vi "K8055.vi"() -> (0 "Numeric":dbl)   [LabVIEW 2012]
uses:
  K8055D.dll
panel:
  in  "Card":dbl
  out "Numeric 2":dbl
  in  "Knob 2":dbl(knob) min=0.0 max=255.0 step=1.0 scale=0.0..255.0
  in  "Knob":dbl(knob) max=255.0 step=1.0 scale=0.0..255.0
  out "Boolean 13":bool
  out "Boolean 12":bool
  out "Boolean 11":bool
  out "Boolean 10":bool
  out "Boolean 9":bool
  in  "Boolean 8":bool
  in  "Boolean 7":bool
  in  "Boolean 6":bool
  in  "Boolean 5":bool
  in  "Boolean 4":bool
  in  "Boolean 3":bool
  in  "Boolean 2":bool
  in  "Boolean":bool
  # "Driver for Velleman K8055 board\nproblems?  email  mike.rendall@gmail.com"
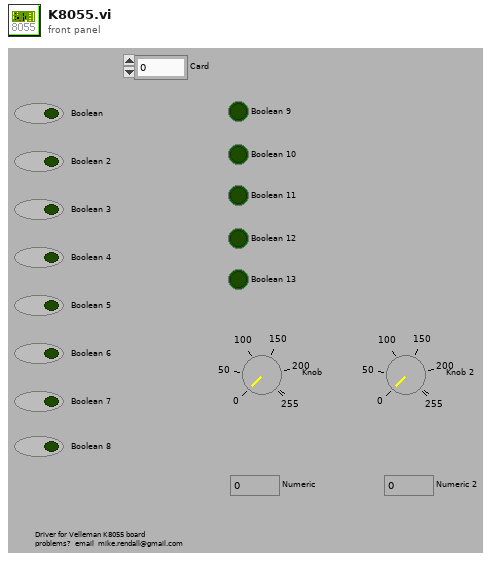
[diagram p1: front panel]
types:
  T1 = cluster{"Boolean array[0]":bool, "Boolean array[1]":bool, "Boolean array[2]":bool, "Boolean array[3]":bool, "Boolean array[4]":bool, "Boolean array[5]":bool, "Boolean array[6]":bool, "Boolean array[7]":bool, "Boolean array[8]":bool}
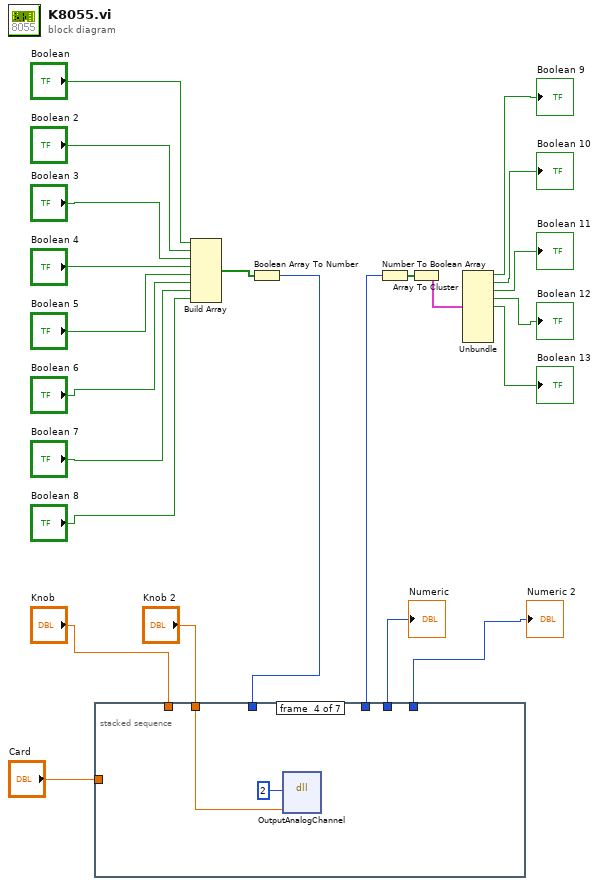
[diagram p0: block diagram]
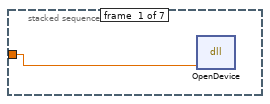
[diagram p2: hidden frame]
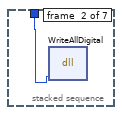
[diagram p3: hidden frame]
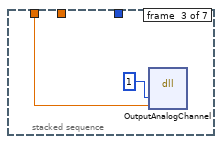
[diagram p4: hidden frame]
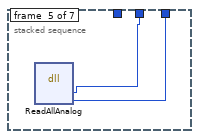
[diagram p5: hidden frame]
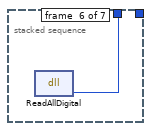
[diagram p6: hidden frame]
diagram:
  n1 = Build Array("Boolean", "Boolean 2", "Boolean 3", "Boolean 4", "Boolean 5", "Boolean 6", "Boolean 7", "Boolean 8") -> (w15:bool[])
  n2 = Boolean Array To Number(Boolean array=w15) -> (number=w13:u32)
  n3 = stacked-sequence {
    tunnel: "Card" -> [w24 _ _ _ _ _ _]
    tunnel: w13 -> [_ w25 _ _ _ _ _]
    tunnel: "Knob" -> [_ _ w27 _ _ _ _]
    tunnel: "Knob 2" -> [_ _ _ w29 _ _ _]
    tunnel: [_ _ _ _ w31 _ _] -> w10
    tunnel: [_ _ _ _ w30 _ _] -> w9
    tunnel: [_ _ _ _ _ w32 _] -> w8
    frame #0 {
      n4 = dll-call lib="C:/Users/edm/Desktop/experiment control/subvis/USB DAQ/K8055D.dll" fn="OpenDevice"(w24) -> ()  [unwired: 5 in, 2 out]
    }
    frame #1 {
      n5 = dll-call lib="C:/Users/edm/Desktop/experiment control/subvis/USB DAQ/K8055D.dll" fn="WriteAllDigital"(w25) -> ()  [unwired: 5 in, 2 out]
    }
    frame #2 {
      n6 = dll-call lib="C:/Users/edm/Desktop/experiment control/subvis/USB DAQ/K8055D.dll" fn="OutputAnalogChannel"(1 ("input param"), w27) -> ()  [unwired: 6 in, 2 out]
    }
    frame #3 {
      n7 = dll-call lib="C:/Users/edm/Desktop/experiment control/subvis/USB DAQ/K8055D.dll" fn="OutputAnalogChannel"(2 ("input param"), w29) -> ()  [unwired: 6 in, 2 out]
    }
    frame #4 {
      n8 = dll-call lib="C:/Users/edm/Desktop/experiment control/subvis/USB DAQ/K8055D.dll" fn="ReadAllAnalog"() -> (w31:i32, w30:i32)  [unwired: 6 in, 2 out]
    }
    frame #5 {
      n9 = dll-call lib="C:/Users/edm/Desktop/experiment control/subvis/USB DAQ/K8055D.dll" fn="ReadAllDigital"() -> (w32:i32)  [unwired: 3 in, 2 out]
    }
    frame #6 {
    }
  }
  "Numeric" <- w10
  "Numeric 2" <- w9
  n10 = Number To Boolean Array(number=w8) -> (Boolean array=w7:bool[])
  n11 = Array To Cluster(array=w7) -> (cluster=w6:T1)
  n12 = Unbundle(w6) -> ("Boolean array[0]"=→"Boolean 9":bool, "Boolean array[1]"=→"Boolean 10":bool, "Boolean array[2]"=→"Boolean 11":bool, "Boolean array[3]"=→"Boolean 12":bool, "Boolean array[4]"=→"Boolean 13":bool)  [unwired: 4 out]
